vi "Unflatten Results STYP.vi"(11 "Result in":string) -> (3 "Result out":T1 {"Status" items=["Service Error"=504, "Abort"=503, "Fail"=500, "Pass"=200]})   [LabVIEW 2014]
uses:
  Controls/Job Results - STYP.ctl
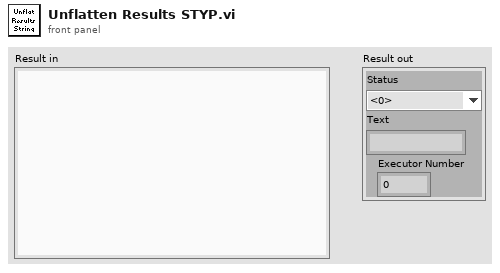
[diagram p1: front panel]
types:
  T1 = typedef "Job Results - STYP.ctl" = cluster{"Status":u16, "Text":string, "Executor Number":i32}
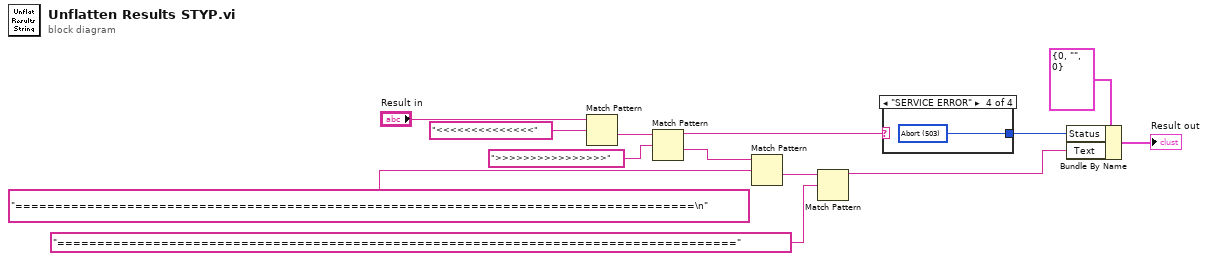
[diagram p0: block diagram]
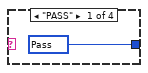
[diagram p2: hidden frame]
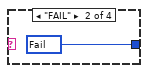
[diagram p3: hidden frame]
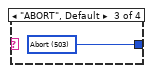
[diagram p4: hidden frame]
diagram:
  n1 = Match Pattern(string="Result in", regular expression="<<<<<<<<<<<<<<" ("format string")) -> (after substring=w8:string)  [unwired: 1 in, 3 out]
  n2 = Match Pattern(string=w8, regular expression=">>>>>>>>>>>>>>>>" ("format string")) -> (before substring=w6:string, after substring=w4:string)  [unwired: 1 in, 2 out]
  n3 = Match Pattern(string=w4, regular expression="=====================================================================================\n" ("format string")) -> (after substring=w5:string)  [unwired: 1 in, 3 out]
  n4 = Match Pattern(string=w5, regular expression="=====================================================================================" ("format string")) -> (before substring=w2:string)  [unwired: 1 in, 3 out]
  n5 = case shown="\"SERVICE ERROR\"" w6 {
    tunnel: [w14 w15 w16 w17] -> w12
    frame "PASS" {
      w14 = u16 200 items=["Service Error"=504, "Abort"=503, "Fail"=500, "Pass"=200] ("Status")
    }
    frame "FAIL" {
      w15 = u16 500 items=["Service Error"=504, "Abort"=503, "Fail"=500, "Pass"=200] ("Status")
    }
    frame "ABORT", Default {
      w16 = u16 503 items=["Service Error"=504, "Abort"=503, "Fail"=500, "Pass"=200] ("Status")
    }
    frame "SERVICE ERROR" {
      w17 = u16 503 items=["Service Error"=504, "Abort"=503, "Fail"=500, "Pass"=200] ("Status")
    }
  }
  n6 = Bundle By Name(cluster=T1 {"Status"=0, "Text"="", "Executor Number"=0} ("Result out"), "Status"=w12, "Text"=w2) -> (→"Result out":T1)
